vi "PickActiveAttackers.vi"(0 "object in":refnum<class "StandardAttackPlay.lvclass">, 2 "AllyRobots":refnum<class "Robot.lvclass">[](array[class]), 4 "AllyTeamIds":T1[](array[typedef]), 5 "error in (no error)":errorcluster) -> (14 "object out":refnum<class "StandardAttackPlay.lvclass">, 16 "ActiveAttackers":refnum<class "Robot.lvclass">[](array[class]), 19 "error out":errorcluster)   [LabVIEW 2023, in "StandardAttackPlay.lvclass"]
uses:
  StandardAttackPlay.lvclass
  Robot_class/Robot.lvclass
  STP_Parameters/AllyTeam.ctl
  StandardAttackPlay.lvclass/StandardAttackPlay.ctl
  Utilities_class/Utilities.lvclass
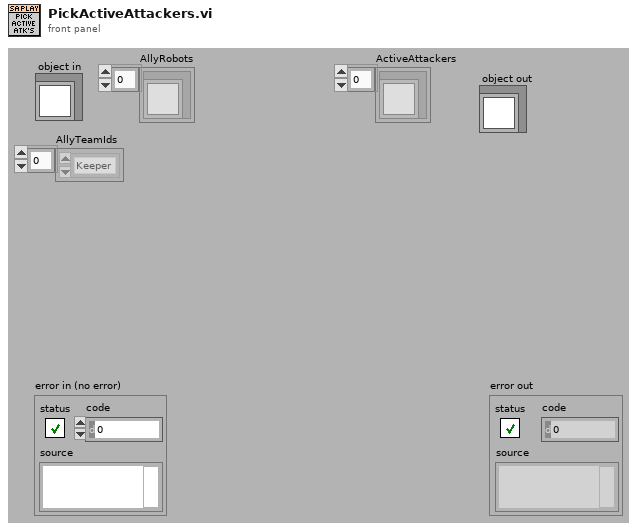
[diagram p1: front panel]
types:
  T1 = typedef "AllyTeam.ctl" = enum16{"Keeper", "Defender", "Attacker"}
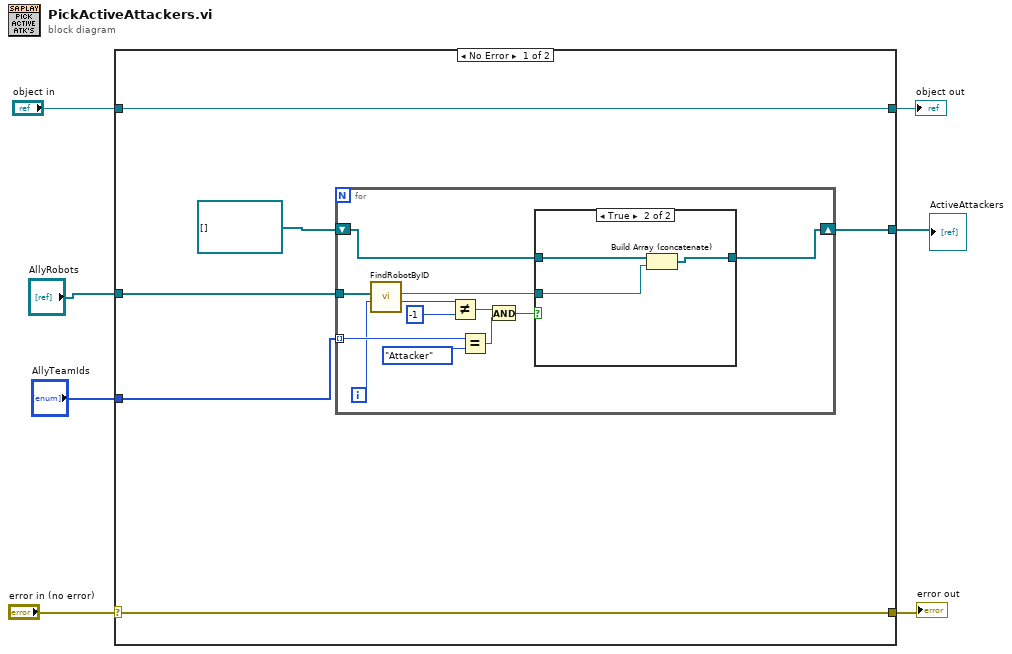
[diagram p0: block diagram]
diagram:
  n1 = case shown="No Error" "error in (no error)" {
    selector: "error in (no error)" -> [w13 w31]
    tunnel: [w13 w31] -> w6
    tunnel: [w12 w30] -> w4
    tunnel: "object in" -> [w12 w30]
    tunnel: [w10 _] -> w3
    tunnel: "AllyRobots" -> [w9 _]
    tunnel: "AllyTeamIds" -> [w8 _]
    frame No Error {
      n2 = for {
        tunnel: w8 -> [w24] mode=indexing
        tunnel: w9 -> [w18]
        shift-right: [w22] -> w10
        shift-left: refnum<class "Robot.lvclass">[] [] ("RobotRef") -> [w23]
        i -> [w19]
        n3 = call "FindRobotByID.vi"("id"=w19, "RobotRef"=w18) -> ("index"=w21:i32, "Robot"=w14:refnum<class "Robot.lvclass">)  [unwired: 6 in, 2 out]
        n4 = Not Equal?(x=w21, y=-1) -> (x != y?=w17:bool)
        n5 = Equal?(x=w24, y=AllyTeam."Attacker" ("AllyTeam")) -> (x = y?=w15:bool)
        n6 = And(x=w17, y=w15) -> (x .and. y?=w16:bool)
        n7 = case shown="True" w16 {
          tunnel: w23 -> [w26 w29]
          tunnel: [w26 w28] -> w22
          tunnel: w14 -> [_ w27]
          frame False {
          }
          frame True {
            n8 = Build Array (concatenate)(w29, w27) -> (w28:refnum<class "Robot.lvclass">[])
          }
        }
      }
    }
    frame Error {
    }
  }
  "error out" <- w6
  "object out" <- w4
  "ActiveAttackers" <- w3
